vi "Read Data.vi"(8 "error in (no error)":errorcluster, 11 "SIM AI Driver in":refnum<class "SIM AI Driver.lvclass">) -> (0 "error out":errorcluster, 2 "Daq Data":T1, 3 "SIM AI Driver out":refnum<class "SIM AI Driver.lvclass">)   [LabVIEW 2022 SP3, in "SIM AI Driver.lvclass"]
uses:
  SIM AI Driver.lvclass
  DAQ Data/AIDAQ Data.ctl
  SIM AI Driver.lvclass/SIM AI Driver.ctl
  <vilib>/numeric/Random Number (Range) DBL.vi
  DAQ Data/AI Daq Data.lvlib
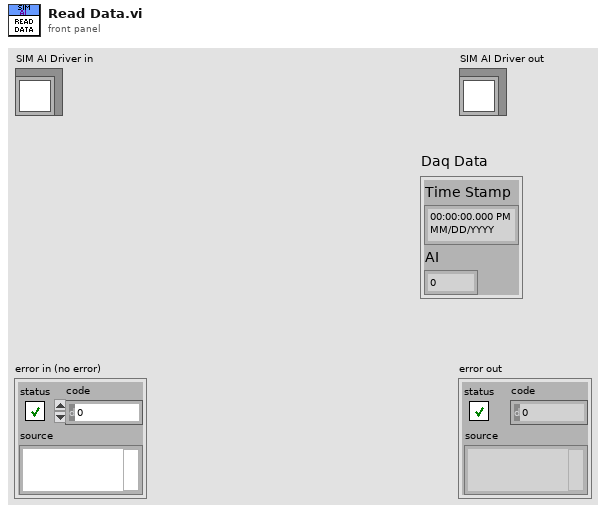
[diagram p1: front panel]
types:
  T1 = typedef "AI Daq Data.lvlib/AIDAQ Data.ctl" = cluster{"Time Stamp":timestamp, "AI":dbl}
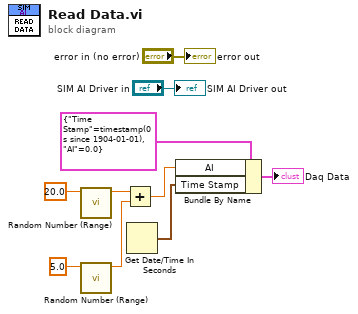
[diagram p0: block diagram]
diagram:
  n1 = call-poly <vilib>:"Random Number (Range).vi"("upper bound (100)"=20.0) -> ("number"=w9:dbl)  [unwired: 10 in]
  n2 = call-poly <vilib>:"Random Number (Range).vi"("upper bound (100)"=5.0) -> ("number"=w6:dbl)  [unwired: 10 in]
  n3 = Add(x=w9, y=w6) -> (x+y=w4:dbl)
  n4 = Get Date/Time In Seconds() -> (seconds since 1Jan1904=w3:timestamp)
  n5 = Bundle By Name(cluster=T1 {"Time Stamp"=timestamp(0 s since 1904-01-01), "AI"=0.0} ("Daq Data"), "AI"=w4, "Time Stamp"=w3) -> (→"Daq Data":T1)
  "error out" <- "error in (no error)"
  "SIM AI Driver out" <- "SIM AI Driver in"
